vi "Adjust ADCs.vi"(0 "Live Raw USB data":u16[](array[numeric]), 1 "Original CalData":dbl[][](array[numeric]), 3 "CustomCal?":bool, 9 "Clear?":bool, 11 "Recal?":bool) -> (4 "LiveData":T1 {"Reference/Temperature 2" format="%.2f"; "Accelerometer" format="%.2f"; "Battery" format="%.2f"; "Reference/Temperature" format="%.2f"; "LoadSensors" format="%.2f"})   [LabVIEW 2013]
uses:
  Controls/LiveData.ctl
  Controls/SignalProcess.ctl
  Controls/Gen2 FT Globals.vi
panel:
  out "transposed array":dbl[][](array[numeric])
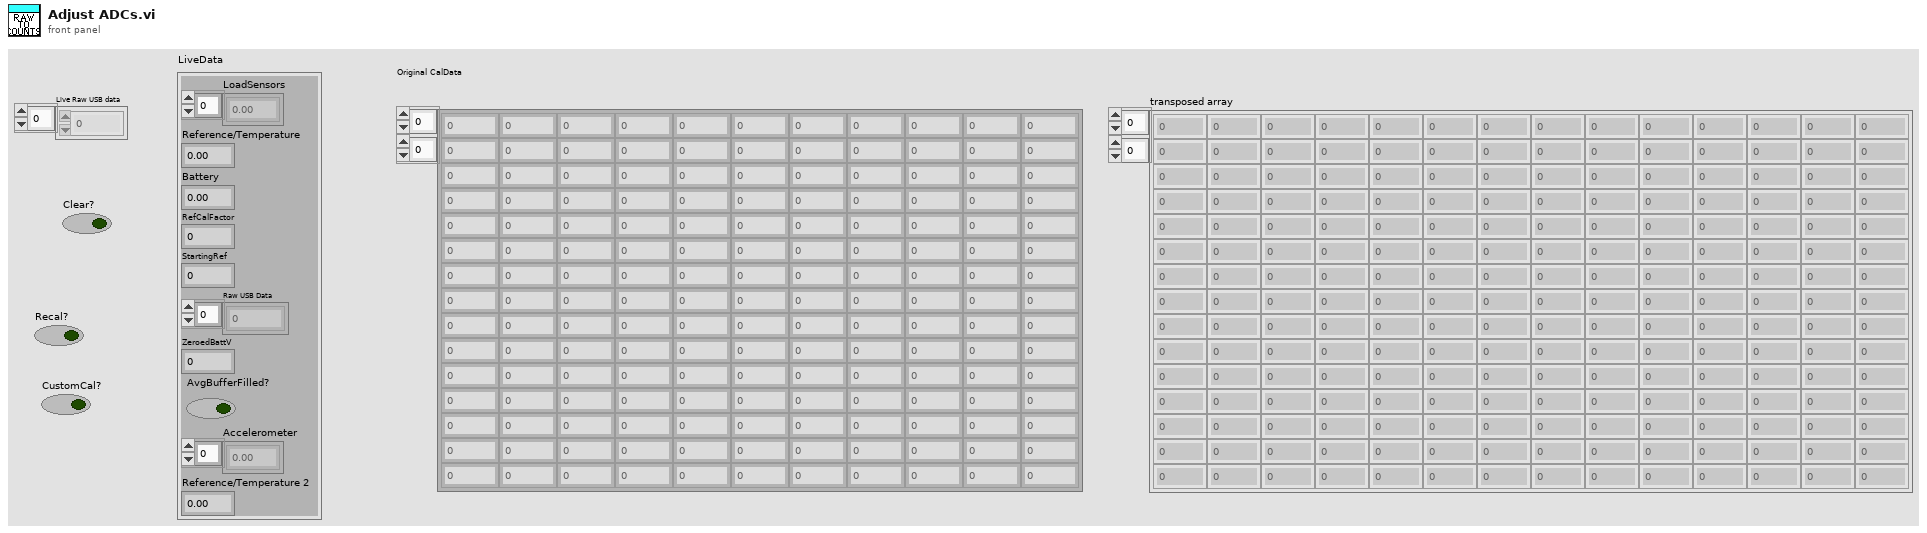
[diagram p1: front panel]
types:
  T1 = typedef "LiveData.ctl" = cluster{"LoadSensors":dbl[], "Reference/Temperature":dbl, "Battery":dbl, "RefCalFactor":dbl, "StartingRef":dbl, "Raw USB Data":u16[], "ZeroedBattV":dbl, "AvgBufferFilled?":bool, "Accelerometer":dbl[], "Reference/Temperature 2":dbl}
  T2 = typedef "SignalProcess.ctl" = enum16{"Remove Duplicates", "Adjust Channels", "Filter Signal", "Fill Average Array", "Recalibrate", "Calibrate Accelerometers", "Adjust Against Ref", "Timeout"}
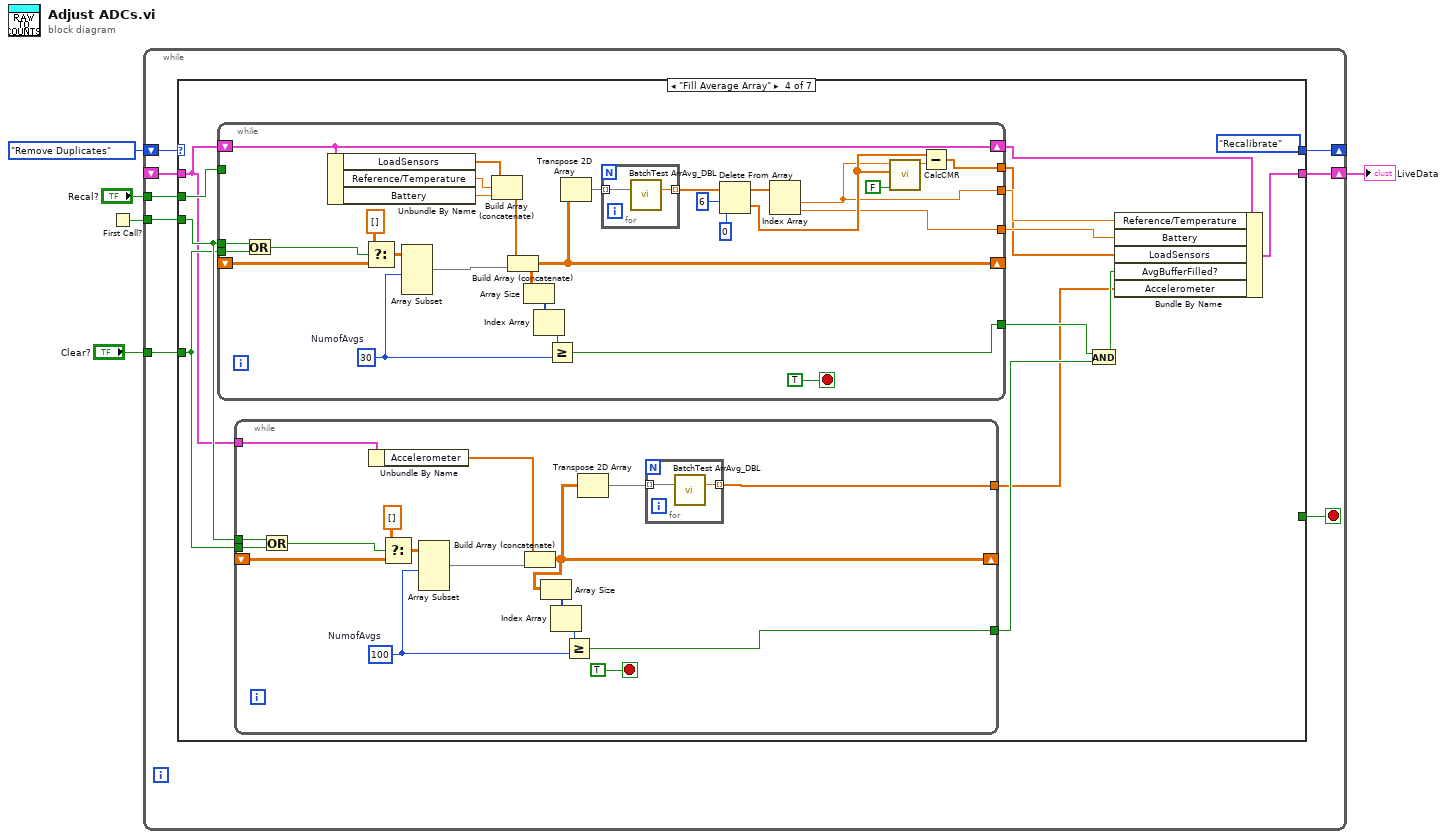
[diagram p0: block diagram]
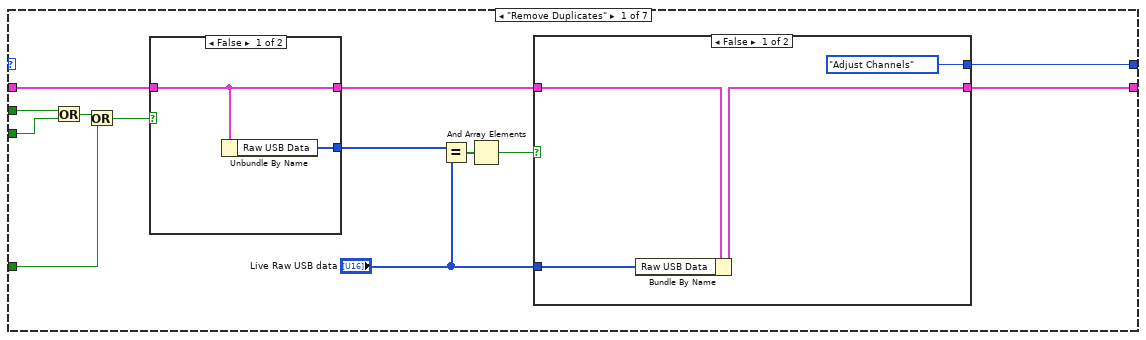
[diagram p2: hidden frame]
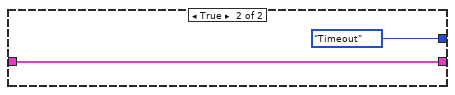
[diagram p3: hidden frame]
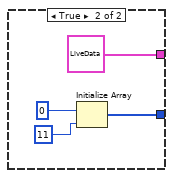
[diagram p4: hidden frame]
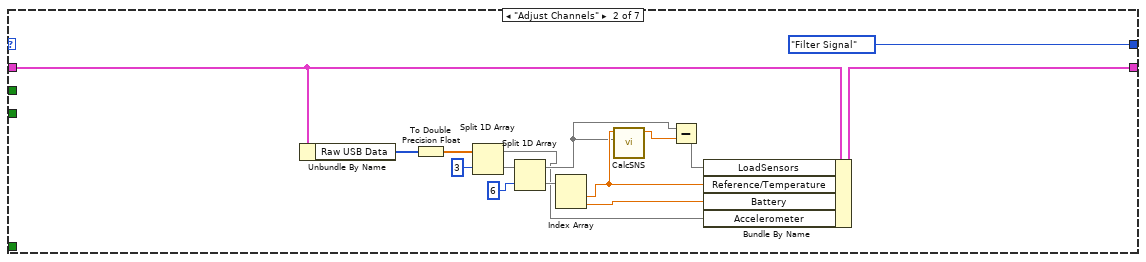
[diagram p5: hidden frame]
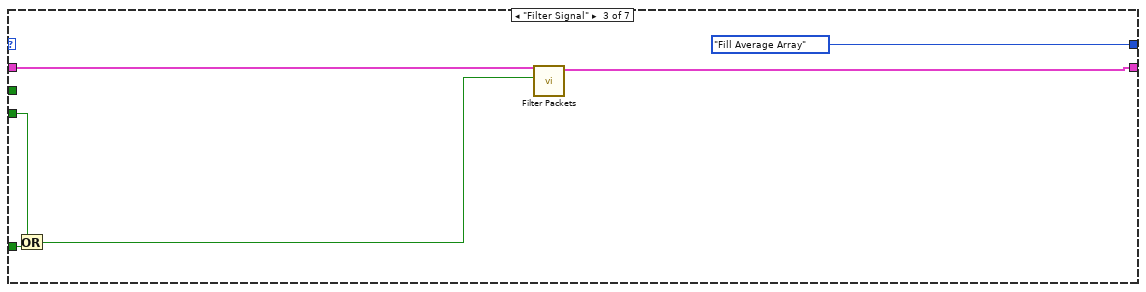
[diagram p6: hidden frame]
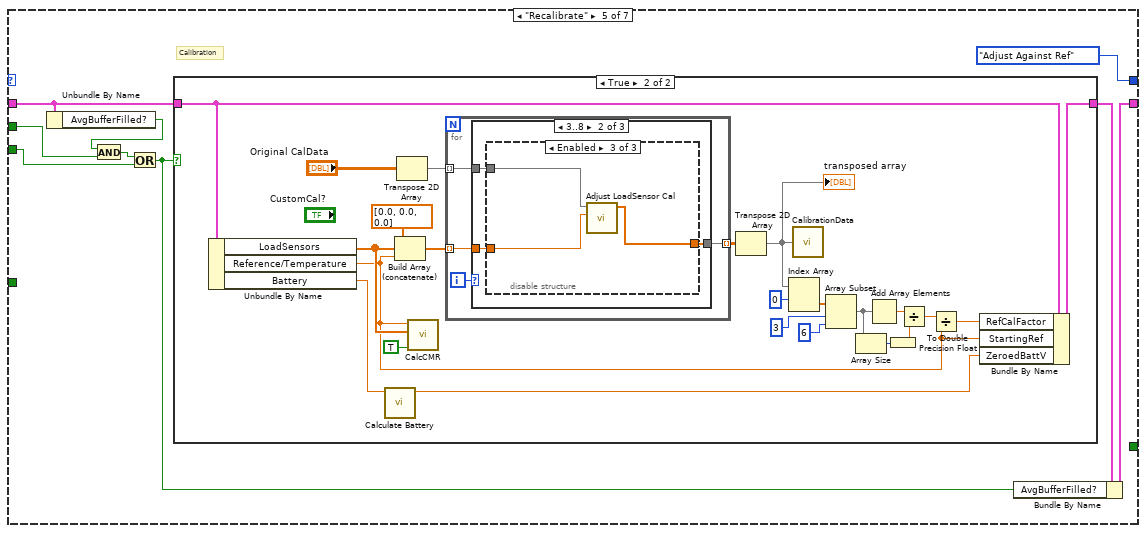
[diagram p7: hidden frame]
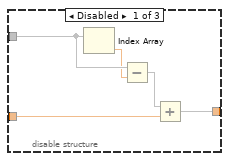
[diagram p10: hidden frame]
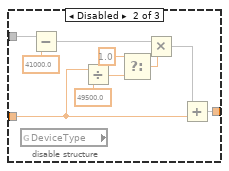
[diagram p11: hidden frame]
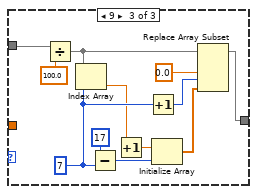
[diagram p12: hidden frame]
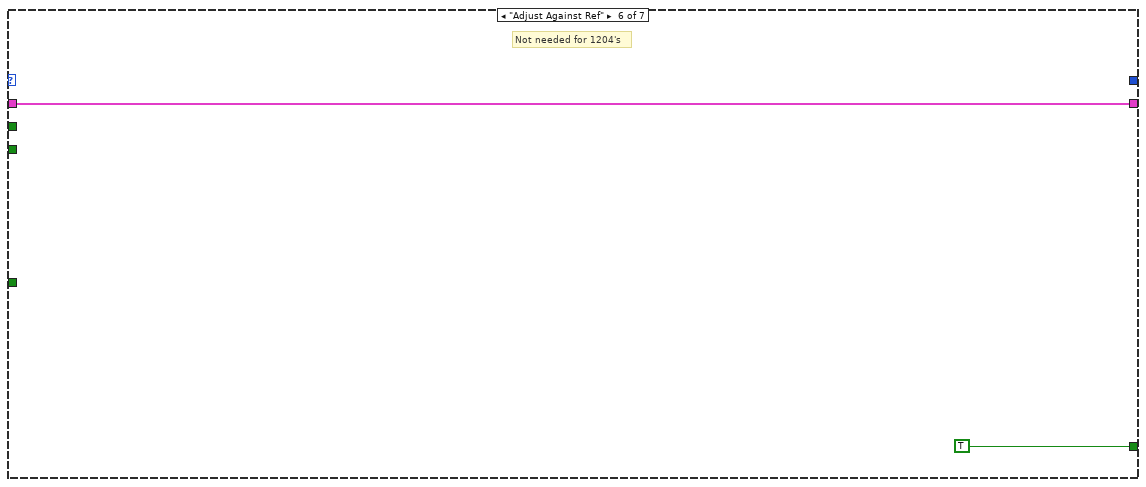
[diagram p13: hidden frame]
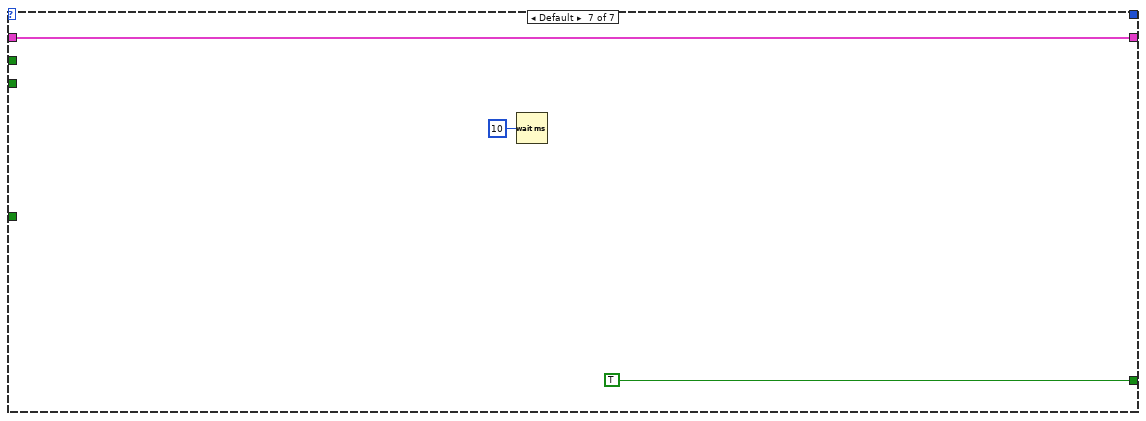
[diagram p14: hidden frame]
diagram:
  n1 = First Call?() -> (First Call?: T/F=w4:bool)
  n2 = while {
    shift-right: [w13] -> w2
    shift-left: _ -> [w10]
    shift-right: [w11] -> _
    shift-left: SignalProcess."Remove Duplicates" -> [w12]
    tunnel: w4 -> [w8]
    tunnel: "Recal?" -> [w7]
    tunnel: "Clear?" -> [w6]
    stop <- w9 stop-if-true
    n3 = case shown="\"Fill Average Array\"" w12 {
      tunnel: [w19 w47 w58 w61 w125 w195 w199] -> w13
      tunnel: [w21 SignalProcess."Filter Signal" SignalProcess."Fill Average Array" SignalProcess."Recalibrate" ("f") SignalProcess."Adjust Against Ref" _ _] -> w11
      tunnel: w10 -> [w26 w48 w59 w69 w127 w195 w199]
      tunnel: [_ _ _ _ _ TRUE TRUE] -> w9
      tunnel: w8 -> [w18 _ w56 w71 w131 _ _]
      tunnel: w7 -> [w25 _ _ w72 w132 _ _]
      tunnel: w6 -> [w14 _ w55 w70 _ _ _]
      frame "Remove Duplicates" {
        n4 = Or(x=w25, y=w18) -> (x .or. y?=w15:bool)
        n5 = Or(x=w15, y=w14) -> (x .or. y?=w16:bool)
        n6 = case shown="False" w16 {
          tunnel: [w34 T1 {"LoadSensors"=[], "Reference/Temperature"=0.0, "Battery"=0.0, "RefCalFactor"=0.0, "StartingRef"=0.0, "Raw USB Data"=[], "ZeroedBattV"=0.0, "AvgBufferFilled?"=FALSE, "Accelerometer"=[], "Reference/Temperature 2"=0.0} ("LiveData")] -> w20
          tunnel: w26 -> [w34 _]
          tunnel: [w33 w36] -> w24
          frame False {
            n7 = Unbundle By Name(w34) -> ("Raw USB Data"=w33:u16[])
          }
          frame True {
            n8 = Initialize Array(u16 0 ("element"), 11 ("dimension size")) -> (w36:u16[])
          }
        }
        n9 = Equal?(x=w24, y="Live Raw USB data") -> (x = y?=w23:bool[])
        n10 = And Array Elements(Boolean array=w23) -> (logical AND=w22:bool)
        n11 = case shown="False" w22 {
          tunnel: [SignalProcess."Adjust Channels" SignalProcess."Timeout"] -> w21
          tunnel: "Live Raw USB data" -> [w27 _]
          tunnel: w20 -> [w29 w31]
          tunnel: [w28 w31] -> w19
          frame False {
            n12 = Bundle By Name(cluster=w29, "Raw USB Data"=w27) -> (w28:T1)
          }
          frame True {
          }
        }
      }
      frame "Adjust Channels" {
        n13 = Unbundle By Name(w48) -> ("Raw USB Data"=w45:u16[])
        n14 = To Double Precision Float(number=w45) -> (double precision float=w44:dbl[])
        n15 = Split 1D Array(array=w44, index=3) -> (first subarray=w39:dbl[], second subarray=w52:dbl[])
        n16 = Split 1D Array(array=w52, index=6) -> (first subarray=w42:dbl[], second subarray=w50:dbl[])
        n17 = Index Array(array=w50) -> (element #1=w43:dbl, element #2=w46:dbl)  [unwired: 2 in]
        n18 = call "CalcSNS.vi"("Load Sensors"=w42, "Ref Sensor"=w43) -> ("delta SNS"=w41:dbl)  [unwired: 9 in]
        n19 = Subtract(x=w42, y=w41) -> (x-y=w40:dbl[])
        n20 = Bundle By Name(cluster=w48, "LoadSensors"=w40, "Reference/Temperature"=w43, "Battery"=w46, "Accelerometer"=w39) -> (w47:T1)
      }
      frame "Filter Signal" {
        n21 = Or(x=w56, y=w55) -> (x .or. y?=w54:bool)
        n22 = call "Filter Packets.vi"("Boolean"=w54, "LiveData in"=w59) -> ("LiveData out"=w58:T1)  [unwired: 9 in]
      }
      frame "Fill Average Array" {
        n23 = while {
          shift-right: [w101] -> _
          shift-left: _ -> [w107]
          shift-right: [w93] -> w60
          shift-left: w69 -> [w93]
          tunnel: w71 -> [w111]
          tunnel: w72 -> [_]
          tunnel: w70 -> [w110]
          tunnel: [w97] -> w68
          tunnel: [w96] -> w67
          tunnel: [w95] -> w66
          tunnel: [w94] -> w63
          stop <- TRUE stop-if-true
          w105 = 30  # NumofAvgs
          n24 = Or(x=w111, y=w110) -> (x .or. y?=w108:bool)
          n25 = Unbundle By Name(w93) -> ("LoadSensors"=w120:dbl[], "Reference/Temperature"=w119:dbl, "Battery"=w118:dbl)
          n26 = Select(t=dbl[][] [], s=w108, f=w107) -> (s? t:f=w106:dbl[][])
          n27 = Array Subset(array=w106, length (row)=w105) -> (w104:dbl[][])  [unwired: 3 in]
          n28 = Build Array (concatenate)(w120, w119, w118) -> (w103:dbl[])
          n29 = Build Array (concatenate)(w103, w104) -> (w101:dbl[][])
          n30 = Array Size(array=w101) -> (size(s)=w114:i32[])
          n31 = Index Array(array=w114) -> (element=w113:i32)  [unwired: 1 in]
          n32 = Greater Or Equal?(x=w113, y=w105) -> (x >= y?=w94:bool)
          n33 = Transpose 2D Array(2D array=w101) -> (transposed array=w102:dbl[][])
          n34 = for {
            tunnel: w102 -> [w123] mode=indexing
            tunnel: [w122] -> w112 mode=indexing
            n35 = call "BatchTest ArrAvg_DBL.vi"("Array In"=w123) -> ("Average"=w122:dbl)  [unwired: 14 in]
          }
          n36 = Delete From Array(array=w112, length=6, index=0) -> (deleted portion=w99:dbl[], array with subset deleted=w115:dbl[])
          n37 = Index Array(array=w115) -> (element #1=w97:dbl, element #2=w96:dbl)  [unwired: 2 in]
          n38 = call "CalcCMR.vi"("Zero?"=FALSE, "Load Sensors"=w99, "Ref Sensor"=w97) -> ("delta SNS"=w100:dbl)  [unwired: 8 in]
          n39 = Subtract(x=w99, y=w100) -> (x-y=w95:dbl[])
        }
        n40 = while {
          shift-right: [w79] -> _
          shift-left: _ -> [w83]
          tunnel: w71 -> [w87]
          tunnel: w70 -> [w86]
          tunnel: w69 -> [w77]
          tunnel: [w76] -> w65
          tunnel: [w75] -> w62
          stop <- TRUE stop-if-true
          w81 = 100  # NumofAvgs
          n41 = Or(x=w87, y=w86) -> (x .or. y?=w84:bool)
          n42 = Unbundle By Name(w77) -> ("Accelerometer"=w78:dbl[])
          n43 = Select(t=dbl[][] [], s=w84, f=w83) -> (s? t:f=w82:dbl[][])
          n44 = Array Subset(array=w82, length (row)=w81) -> (w80:dbl[][])  [unwired: 3 in]
          n45 = Build Array (concatenate)(w78, w80) -> (w79:dbl[][])
          n46 = Array Size(array=w79) -> (size(s)=w89:i32[])
          n47 = Index Array(array=w89) -> (element=w88:i32)  [unwired: 1 in]
          n48 = Greater Or Equal?(x=w88, y=w81) -> (x >= y?=w76:bool)
          n49 = Transpose 2D Array(2D array=w79) -> (transposed array=w74:dbl[][])
          n50 = for {
            tunnel: w74 -> [w92] mode=indexing
            tunnel: [w91] -> w75 mode=indexing
            n51 = call "BatchTest ArrAvg_DBL.vi"("Array In"=w92) -> ("Average"=w91:dbl)  [unwired: 14 in]
          }
        }
        n52 = And(x=w63, y=w65) -> (x .and. y?=w64:bool)
        n53 = Bundle By Name(cluster=w60, "Reference/Temperature"=w68, "Battery"=w67, "LoadSensors"=w66, "AvgBufferFilled?"=w64, "Accelerometer"=w62) -> (w61:T1)
      }
      frame "Recalibrate" {
        # "Calibration"
        n54 = Unbundle By Name(w127) -> ("AvgBufferFilled?"=w126:bool)
        n55 = And(x=w126, y=w132) -> (x .and. y?=w128:bool)
        n56 = Or(x=w128, y=w131) -> (x .or. y?=w124:bool)
        n57 = case shown="True" w124 {
          tunnel: w127 -> [w133 w147]
          tunnel: [w133 w142] -> w129
          frame False {
          }
          frame True {
            n58 = Unbundle By Name(w147) -> ("LoadSensors"=w136:dbl[], "Reference/Temperature"=w135:dbl, "Battery"=w143:dbl)
            n59 = call "Calculate Battery.vi"("Battery A/D in"=w143) -> ("Battery Volts Out"=w141:dbl)  [unwired: 10 in]
            n60 = Build Array (concatenate)(dbl[] [0.0, 0.0, 0.0], w136, w135) -> (w139:dbl[])
            n61 = Transpose 2D Array(2D array="Original CalData") -> (transposed array=w140:dbl[][])
            n62 = call "CalcCMR.vi"("Zero?"=TRUE, "Load Sensors"=w136, "Ref Sensor"=w135) -> ()  [unwired: 8 in, 1 out]
            n63 = for {
              tunnel: w140 -> [w160] mode=indexing
              tunnel: w139 -> [w157] mode=indexing
              tunnel: [w159] -> w137 mode=indexing
              i -> [w158]
              n64 = case shown="3..8" w158 {
                tunnel: w157 -> [_ w163 _]
                tunnel: w160 -> [w161 w164 w188]
                tunnel: [w161 w162 w190] -> w159
                frame Default {
                }
                frame 3..8 {
                  n65 = disable-structure shown="Enabled" {
                    disable-tunnel: w164 -> [w169 w179 w182]
                    disable-tunnel: w163 -> [w166 w170 w180]
                    disable-tunnel: [w165 w177 w181] -> w162
                    frame Disabled {
                      n66 = Index Array(array=w169) -> (element=w168:dbl)  [unwired: 1 in]
                      n67 = Subtract(x=w169, y=w168) -> (x-y=w167:dbl[])
                      n68 = Add(x=w167, y=w166) -> (x+y=w165:dbl[])
                    }
                    frame Disabled {
                      n69 = global read "Gen2 FT Globals.vi" "DeviceType"() -> ()  [unwired: 1 out]
                      n70 = Subtract(x=w179, y=41000.0 ("element")) -> (x-y=w178:dbl[])
                      n71 = Divide(x=w170, y=49500.0) -> (x/y=w172:dbl)
                      n72 = Select(t=1.0, f=w172) -> (s? t:f=w171:dbl)  [unwired: 1 in]
                      n73 = Multiply(x=w178, y=w171) -> (x*y=w175:dbl[])
                      n74 = Add(x=w175, y=w170) -> (x+y=w177:dbl[])
                    }
                    frame Enabled {
                      n75 = call "Adjust LoadSensor Cal.vi"("0_Load"=w180, "LS CalData In"=w182) -> ("LS CalData Out"=w181:dbl[])  [unwired: 9 in]
                    }
                  }
                }
                frame 9 {
                  w186 = 7 ("index of element")
                  n76 = Divide(x=w188, y=100.0) -> (x/y=w183:dbl[])
                  n77 = Index Array(array=w183, index=w186) -> (element=w184:dbl)
                  n78 = Subtract(x=17 ("dimension size"), y=w186) -> (x-y=w193:i32)
                  n79 = Increment(x=w184) -> (x+1=w194:dbl)
                  n80 = Increment(x=w186) -> (x+1=w185:i32)
                  n81 = Initialize Array(w194, w193) -> (w187:dbl[])
                  n82 = Replace Array Subset(array=w183, new element #1=0.0 ("new element/subarray"), new element #2=w187, index #2=w185) -> (w190:dbl[])  [unwired: 1 in]
                }
              }
            }
            n83 = Transpose 2D Array(2D array=w137) -> (transposed array=w146:dbl[][])
            "transposed array" <- w146
            n84 = Index Array(array=w146, index (row)=0) -> (element=w149:dbl[])  [unwired: 1 in]
            n85 = call "CalibrationData.vi"("CalData In"=w146) -> ()  [unwired: 1 out]
            n86 = Array Subset(array=w149, index=3, length=6) -> (w150:dbl[])
            n87 = Array Size(array=w150) -> (size(s)=w152:i32)
            n88 = Add Array Elements(numeric array=w150) -> (sum=w153:dbl)
            n89 = To Double Precision Float(number=w152) -> (double precision float=w151:dbl)
            n90 = Divide(x=w153, y=w151) -> (x/y=w148:dbl)
            n91 = Divide(x=w148, y=w135) -> (x/y=w144:dbl)
            n92 = Bundle By Name(cluster=w147, "RefCalFactor"=w144, "StartingRef"=w135, "ZeroedBattV"=w141) -> (w142:T1)
          }
        }
        n93 = Bundle By Name(cluster=w129, "AvgBufferFilled?"=w124) -> (w125:T1)
      }
      frame "Adjust Against Ref" {
        # "Not needed for 1204's"
      }
      frame Default {
        n94 = Wait (ms)(milliseconds to wait=u32 10) -> ()  [unwired: 1 out]
      }
    }
  }
  "LiveData" <- w2
